vi "Actor Core.vi"(8 "error in":errorcluster, 11 "Cooler":refnum<class "Cooler.lvclass">) -> (0 "error out":errorcluster, 3 "Actor out":refnum<class "Actor.lvclass">)   [LabVIEW 2012, in "Cooler.lvlib" / "Cooler.lvclass"]
doc: "This is Actor Core.vi, the main message handling loop for Actors. An actor usually just sits in this loop and processes messages as they arrive. Any error returned by the message Do.vi call will stop the loop, with error code 43 as the cannonical signal to stop with no error sent to caller. Descendants may override that in Handle Error.vi."
uses:
  Cooler.lvclass
  <vilib>/ActorFramework/Actor/Actor.lvclass
  Dual Controller/Dual Fan/Dual Fan.lvclass
  Water Level/Water Level.lvclass
  <vilib>/ActorFramework/Actor/Actor.lvclass/Actor.ctl
  <vilib>/ActorFramework/Message Enqueuer/Message Enqueuer.lvclass/Message Enqueuer.ctl
  Cooler.lvclass/Cooler.ctl
  Level Controller/Level Controller/Level Controller.lvclass
  <vilib>/ActorFramework/Message Enqueuer/Init from Existing Queue.vi
  <vilib>/ActorFramework/Message Enqueuer/Message Enqueuer.lvclass
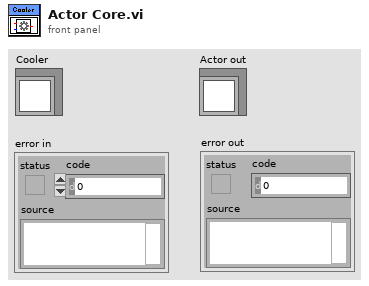
[diagram p1: front panel]
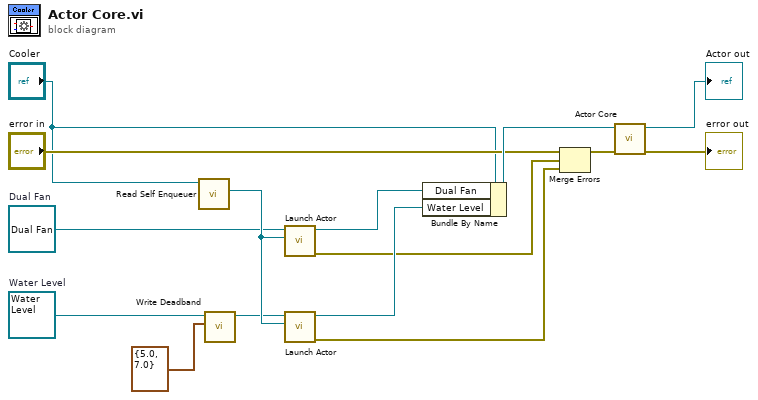
[diagram p0: block diagram]
diagram:
  w6 = refnum<class "Water Level.lvclass"> refnum  # Water Level
  w11 = refnum<class "Dual Fan.lvclass"> refnum  # Dual Fan
  n1 = call <vilib>:"Read Self Enqueuer.vi"("Actor"="Cooler") -> ("Self Enqueuer"=w13:refnum<class "Message Enqueuer.lvclass">)  [unwired: 10 in]
  n2 = call "Write Deadband.vi"("Deadband"=cluster{"LO":dbl, "HI":dbl} {"LO"=5.0, "HI"=7.0}, "Level Controller in"=w6) -> ("Level Controller out"=w5:refnum<class "Water Level.lvclass">)  [unwired: 8 in, 1 out]
  n3 = call <vilib>:"Launch Actor.vi"("Actor-to-Caller Enqueuer"=w13, "Actor"=w11) -> ("error out"=w9:errorcluster, "Caller-To-Actor Enqueuer"=w12:refnum<class "Message Enqueuer.lvclass">)  [unwired: 8 in]
  n4 = call <vilib>:"Launch Actor.vi"("Actor-to-Caller Enqueuer"=w13, "Actor"=w5) -> ("error out"=w8:errorcluster, "Caller-To-Actor Enqueuer"=w14:refnum<class "Message Enqueuer.lvclass">)  [unwired: 8 in]
  n5 = Bundle By Name(cluster="Cooler", "Dual Fan"=w12, "Water Level"=w14) -> (w10:refnum<class "Cooler.lvclass">)
  n6 = Merge Errors("error in", w9, w8) -> (w3:errorcluster)
  n7 = call-parent "Actor Core.vi"("error in"=w3, "Timed Loop Controller"=w10) -> ("error out"=→"error out":errorcluster, "Actor out"=→"Actor out":refnum<class "Actor.lvclass">)  [unwired: 8 in]
